vi "I2C Mux and Digipots.vi"() -> ()   [LabVIEW 2020, in "CTI-Scratchpad.lvlib"]
uses:
  CTI-Scratchpad.lvlib
  CTI/Identity.ctl
  CTI/Error Reporting.ctl
  CTI/GPIO Number.ctl
  CTI/I2C Number.ctl
  CTI/Session/Session.lvclass
  CTI-Peripheral/Multiplexer/TCA9548A I2C Multiplexer/TCA9548A I2C Multiplexer.lvclass
  CTI-Peripheral/Analog Output/Potentiometer I2C/MCP4018 Digipot/MCP4018 Digipot.lvclass
  CTI/VisaComms/VisaComms.lvclass
  CTI/CTI.lvlib
panel:
  in  "Pot (0-127)":u8(slide) scale=0.0..127.0
  in  "I2C7":bool
  in  "I2C6":bool
  in  "I2C5":bool
  in  "I2C4":bool
  in  "Default Address":u8=112 format="%.0x"
  in  "Stop":bool
  in  "I2C3":bool
  in  "I2C2":bool
  in  "I2C1":bool
  in  "I2C0":bool
  out "loop":i32
  out "Identity":T1
  in  "Grove Connector":enum16{"I2C0", "I2C1"}(ring)
  out "error out":errorcluster
  in  "Port":refnum<visa-resource-name>="COM4"
  # "I2C0"
  # "I2C1"
  # "I2C2"
  # "I2C3"
  # "I2C4"
  # "I2C5"
  # "I2C6"
  # "I2C7"
  # "https://wiki.seeedstudio.com/Grove-8-Channel-I2C-Multiplexer-I2C-Hub-TCA9548A/"
  # "https://docs.soldered.com/digipot/overview/"
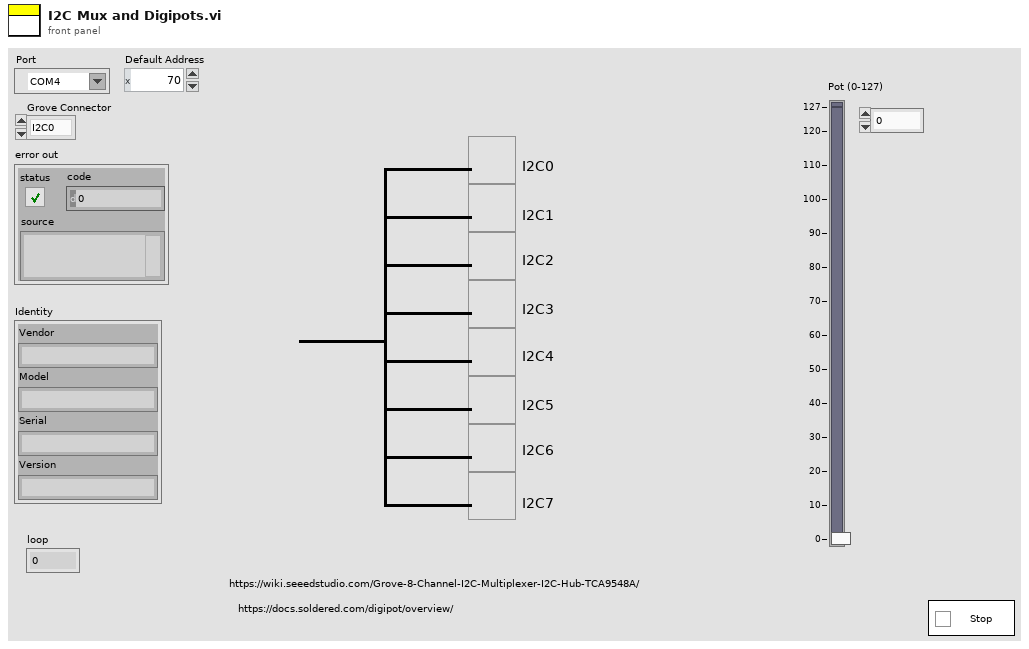
[diagram p1: front panel]
types:
  T1 = typedef "CTI.lvlib/Identity.ctl" = cluster{"Vendor":string, "Model":string, "Serial":string, "Version":string}
  T2 = typedef "CTI.lvlib/Error Reporting.ctl" = enum16{"Minimal", "Moderate", "Full"}
  T3 = typedef "CTI.lvlib/I2C Number.ctl" = i8
  T4 = typedef "CTI.lvlib/GPIO Number.ctl" = i8
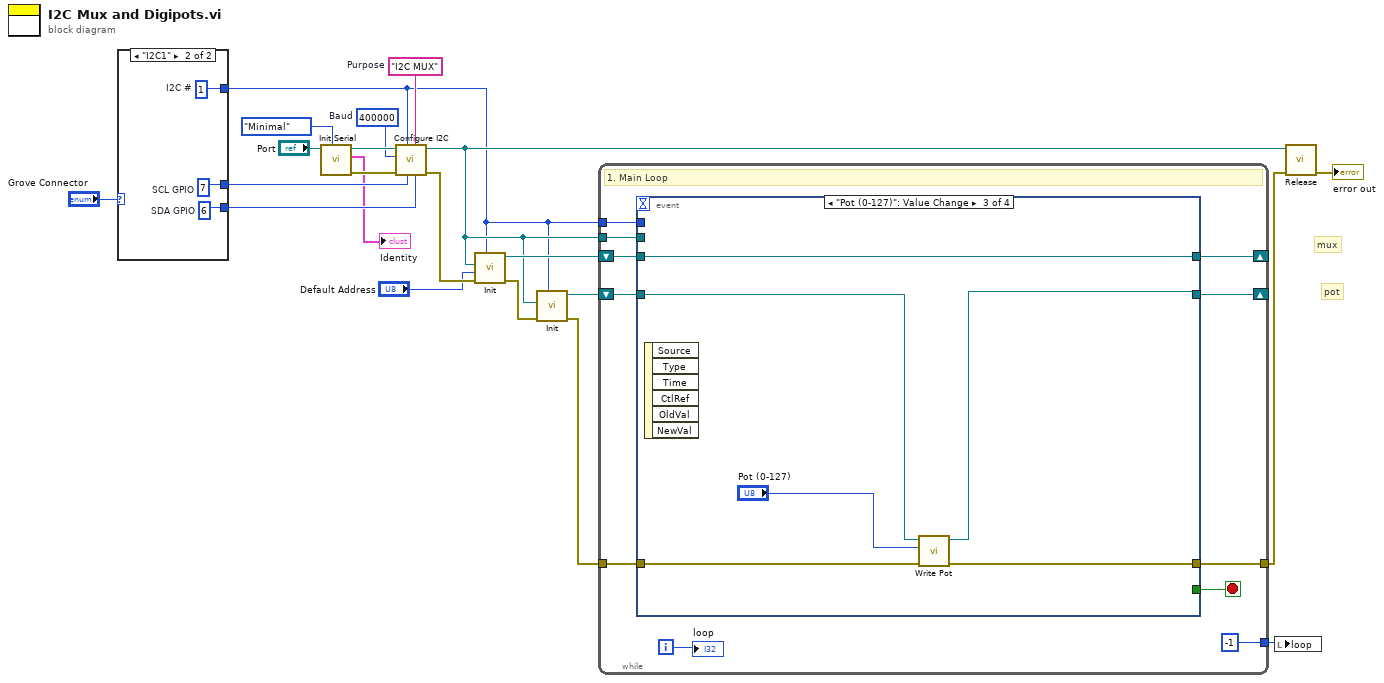
[diagram p0: block diagram]
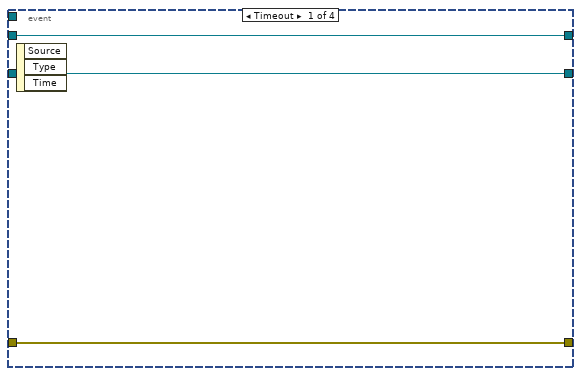
[diagram p2: hidden frame]
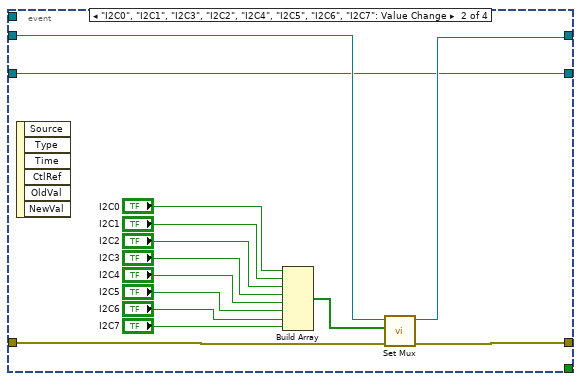
[diagram p3: hidden frame]
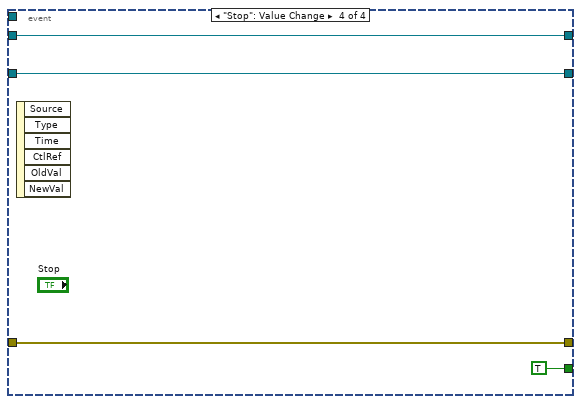
[diagram p4: hidden frame]
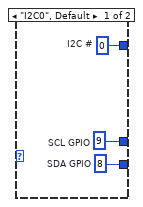
[diagram p5: hidden frame]
diagram:
  w16 = "I2C MUX"  # Purpose
  w17 = u32 400000  # Baud
  # "pot"
  # "mux"
  n1 = case shown="\"I2C1\"" "Grove Connector" {
    tunnel: [w24 w27] -> w14
    tunnel: [w23 w26] -> w13
    tunnel: [w22 w25] -> w1
    frame "I2C0", Default {
      w22 = T3 0  # I2C #
      w23 = T4 8  # SDA GPIO
      w24 = T4 9  # SCL GPIO
    }
    frame "I2C1" {
      w25 = T3 1  # I2C #
      w26 = T4 6  # SDA GPIO
      w27 = T4 7  # SCL GPIO
    }
  }
  n2 = call "Init Serial.vi"("Error Checking (Full)"=Error_Reporting."Minimal", "VISA resource name in"="Port") -> ("error out"=w18:errorcluster, "Identity"=→"Identity":T1, "Session"=w19:refnum<class "Session.lvclass">)  [unwired: 7 in]
  n3 = call "Configure I2C.vi"("SDA GPIO"=w13, "Purpose (\"I2C\")"=w16, "SCL GPIO"=w14, "I2C #"=w1, "error in (no error)"=w18, "Baud"=w17, "Session in"=w19) -> ("error out"=w9:errorcluster, "Session out"=w2:refnum<class "Session.lvclass">)  [unwired: 3 in]
  n4 = call "Init.vi"("I2C #"=w1, "error in (no error)"=w9, "Address"="Default Address", "Session In"=w2) -> ("error out"=w5:errorcluster, "TCA9548A Mux Out"=w8:refnum<class "TCA9548A I2C Multiplexer.lvclass">)  [unwired: 6 in]
  n5 = call "Init.vi"("I2C #"=w1, "error in (no error)"=w5, "Session In"=w2) -> ("error out"=w4:errorcluster, "MCP4018 Digipot Out"=w3:refnum<class "MCP4018 Digipot.lvclass">)  [unwired: 7 in]
  n6 = while {
    tunnel: w4 -> [w37]
    tunnel: [w35] -> w11
    tunnel: [-1] -> w7
    shift-right: [w32] -> _
    shift-left: w8 -> [w38]
    tunnel: w1 -> [w31]
    tunnel: w2 -> [w30]
    shift-right: [w28] -> _
    shift-left: w3 -> [w29]
    i -> [w36]
    stop <- w34 stop-if-true
    # "1. Main Loop"
    n7 = event shown="[2] \"Pot (0-127)\": Value Change" {
      selector: _ -> [_ _ _ _]
      dyn-events: _ -> [_ _ _ _]
      timeout: _ -> [_ _ _ _]
      tunnel: w38 -> [w40 w53 w61 w63]
      tunnel: w37 -> [w41 w55 w60 w64]
      tunnel: [w41 w54 w56 w64] -> w35
      tunnel: [_ _ _ TRUE] -> w34
      tunnel: [w40 w52 w61 w63] -> w32
      tunnel: w31 -> [_ _ _ _]
      tunnel: w30 -> [_ _ _ _]
      tunnel: w29 -> [w39 w42 w58 w62]
      tunnel: [w39 w42 w57 w62] -> w28
      event Timeout {
        n8 = event-data() -> ()  [unwired: 1 in, 3 out]
      }
      event "I2C0", "I2C1", "I2C3", "I2C2", "I2C4", "I2C5", "I2C6", "I2C7": Value Change {
        n9 = event-data() -> ()  [unwired: 1 in, 6 out]
        n10 = Build Array("I2C0", "I2C1", "I2C2", "I2C3", "I2C4", "I2C5", "I2C6", "I2C7") -> (w51:bool[])
        n11 = call-dynamic "Set Mux.vi"("error in (no error)"=w55, "Mux Enabled Channels"=w51, "TCA9548A Mux in"=w53) -> ("error out"=w54:errorcluster, "TCA9548A Mux out"=w52:refnum<class "TCA9548A I2C Multiplexer.lvclass">)  [unwired: 7 in]
      }
      event "Pot (0-127)": Value Change {
        n12 = event-data() -> ()  [unwired: 1 in, 6 out]
        n13 = call-dynamic "Write Pot.vi"("error in (no error)"=w60, "Pot Value(0-127)"="Pot (0-127)", "MCP4018 Digipot in"=w58) -> ("error out"=w56:errorcluster, "MCP4018 Digipot out"=w57:refnum<class "MCP4018 Digipot.lvclass">)  [unwired: 7 in]
      }
      event "Stop": Value Change {
        n14 = event-data() -> ()  [unwired: 1 in, 6 out]
      }
    }
    "loop" <- w36
  }
  n15 = local write "loop"(w7) -> ()
  n16 = call-dynamic "Release.vi"("error in (no error)"=w11, "Session in"=w2) -> ("error out"=→"error out":errorcluster)  [unwired: 9 in]
